vi "main.vi"() -> ()   [LabVIEW 2019]
panel:
  out "Equation":string
  out "NormalVector":dbl[](array[numeric])
  out "D":dbl
  out "Three Points":dbl[][](array[numeric])
  out "Position":dbl[](array[numeric])
  in  "Zaxis Step Size":dbl
  out "SytemID":i32
  out "AxisID":string[](array[string])
  out "Ready":bool
  in  "stop":bool
  out "Error Out":errorcluster
  out "SetYPosition":dbl
  out "SetXPosition":dbl
  # "Ax + By + Cz = <A,B,C> . <X_0,Y_0,Z_0> = D"
  # "A"
  # "B"
  # "C"
  # "X"
  # "Y"
  # "Z"
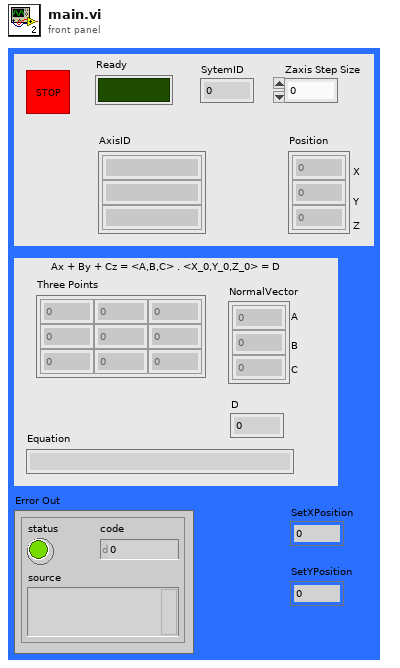
[diagram p1: front panel]
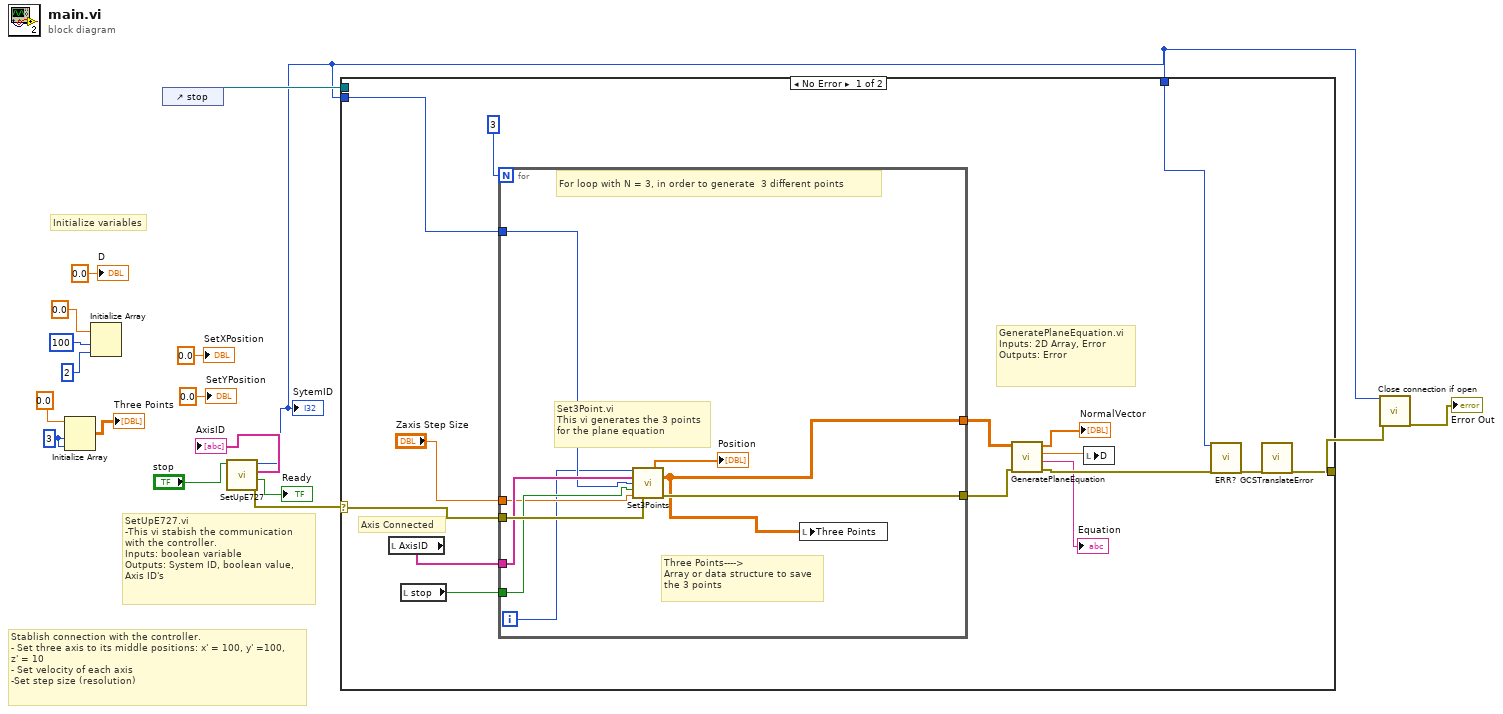
[diagram p0: block diagram]
diagram:
  w9 = 3 ("dimension size")
  # "SetUpE727.vi\n-This vi stabish the communication \nwith the controller.\nInputs: boolean variable\nOutputs: System ID, boolean value,\nAxis ID's"
  # "Initialize variables"
  # "Stablish connection with the controller.\n- Set three axis to its middle positions: x' = 100, y' =100, \nz' = 10\n- Set velocity of each axis\n-Set step size (resolution)"
  n1 = Initialize Array(0.0 ("element"), w9, w9) -> (→"Three Points":dbl[][])
  n2 = Initialize Array(0.0 ("element"), 100 ("dimension size"), 2 ("dimension size")) -> ()  [unwired: 1 out]
  n3 = control-ref of="stop"() -> (w16:refnum<vi>)
  n4 = call "SetUpE727.vi"("stop"="stop") -> ("Error Out"=w1:errorcluster, "Redy"=→"Ready":bool, "Axis ID´s"=→"AxisID":string[], "SystemID"=w3:i32)  [unwired: 7 in]
  "SytemID" <- w3
  n5 = case shown="No Error" w1 {
    selector: w1 -> [w32 w42]
    tunnel: w3 -> [w31 _]
    tunnel: w16 -> [_ _]
    tunnel: w3 -> [w24 _]
    tunnel: [w25 w42] -> w6
    frame No Error {
      # "GeneratePlaneEquation.vi\nInputs: 2D Array, Error\nOutputs: Error"
      # "Axis Connected"
      n6 = local read "AxisID"() -> (w30:string[])
      n7 = local read "stop"() -> (w29:bool)
      n8 = for {
        N: 3 -> [_]
        tunnel: w31 -> [w37]
        tunnel: w32 -> [w41]
        tunnel: w30 -> [w40]
        tunnel: w29 -> [w39]
        tunnel: "Zaxis Step Size" -> [w38]
        tunnel: [w36] -> w23
        tunnel: [w35] -> w22
        i -> [w33]
        # "Three Points---->\nArray or data structure to save\nthe 3 points"
        # "For loop with N = 3, in order to generate  3 different points"
        # "Set3Point.vi\nThis vi generates the 3 points\nfor the plane equation"
        n9 = call "Set3Points.vi"("Counter"=w33, "axis id"=w40, "System number"=w37, "stop"=w39, "Z Axis Step  Size"=w38, "Error In"=w41) -> ("Relative Position"=→"Position":dbl[], "3Points2DArray"=w35:dbl[][], "Error Out"=w36:errorcluster)  [unwired: 7 in]
        n10 = local write "Three Points"(w35) -> ()
      }
      n11 = call "GeneratePlaneEquation.vi"("Error In"=w23, "Three  points"=w22) -> ("Error Out"=w21:errorcluster, "Equation"=→"Equation":string, "D"=w19:dbl, "NormalVector"=→"NormalVector":dbl[])  [unwired: 6 in]
      n12 = local write "D"(w19) -> ()
      n13 = call "ERR?.vi"("System no."=w24, "error in"=w21) -> ("error out"=w28:errorcluster)  [unwired: 17 out]
      n14 = call "GCSTranslateError.vi"("error in"=w28) -> ("error out"=w25:errorcluster)  [unwired: 18 out]
    }
    frame Error {
    }
  }
  n15 = call "Close connection if open.vi"("System no."=w3, "error in"=w6) -> ("error out"=→"Error Out":errorcluster)  [unwired: 1 in, 16 out]
  "D" <- 0.0 ("D")
  "SetXPosition" <- 0.0 ("SetXPosition")
  "SetYPosition" <- 0.0 ("SetYPosition")
